vi "CC Past Noon Check.vi"(8 "error in (no error)":errorcluster) -> (0 "error out":errorcluster, 3 "Passed noon":bool)   [LabVIEW 2021]
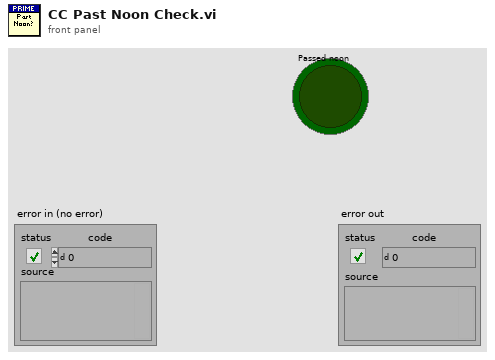
[diagram p1: front panel]
types:
  T1 = typedef "LVDateTimeRec.ctl" = cluster{"fractional second":dbl, "second":i32, "minute":i32, "hour":i32, "day of month":i32, "month":i32, "year":i32, "day of week":i32, "day of year":i32, "DST":i32}
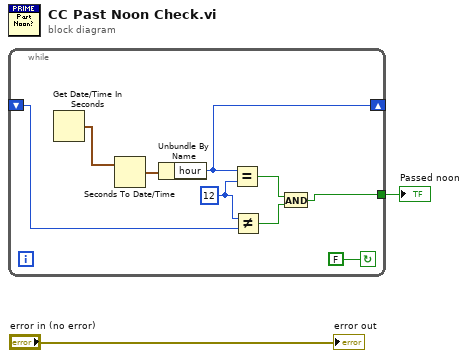
[diagram p0: block diagram]
diagram:
  n1 = while {
    shift-right: [w10] -> _
    shift-left: _ -> [w8]
    tunnel: [w4] -> w1
    stop <- FALSE continue-if-true
    w9 = 12 ("y")
    n2 = Get Date/Time In Seconds() -> (seconds since 1Jan1904=w3:timestamp)
    n3 = Seconds To Date/Time(time stamp (now)=w3) -> (date time rec=w11:T1)  [unwired: 1 in]
    n4 = Unbundle By Name(w11) -> ("hour"=w10:i32)
    n5 = Equal?(x=w10, y=w9) -> (x = y?=w6:bool)
    n6 = Not Equal?(x=w9, y=w8) -> (x != y?=w5:bool)
    n7 = And(x=w6, y=w5) -> (x .and. y?=w4:bool)
  }
  "Passed noon" <- w1
  "error out" <- "error in (no error)"
